vi "Untitled 2.vi"() -> ()   [LabVIEW 2017]
uses:
  JSONtext.lvlib
panel:
  out "Variant out":variant
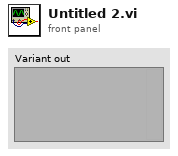
[diagram p1: front panel]
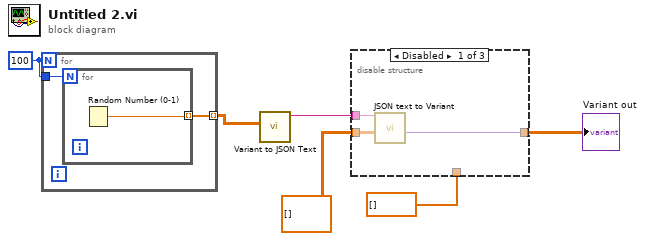
[diagram p0: block diagram]
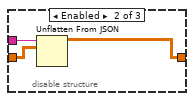
[diagram p2: hidden frame]
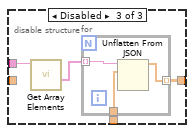
[diagram p3: hidden frame]
diagram:
  w2 = 100
  n1 = for {
    N: w2 -> [_]
    tunnel: [w8] -> w6 mode=indexing
    tunnel: w2 -> [w7]
    n2 = for {
      N: w7 -> [_]
      tunnel: [w9] -> w8 mode=indexing
      n3 = Random Number (0-1)() -> (number: 0 to 1=w9:dbl)
    }
  }
  n4 = call "Variant to JSON Text.vi"("Variant"=w6) -> ("<JSON>"=w5:string)  [unwired: 8 in, 2 out]
  n5 = disable-structure shown="Disabled" {
    disable-tunnel: w5 -> [w12 w15 w19]
    disable-tunnel: dbl[][] [] -> [w11 w14 _]
    disable-tunnel: [w10 w13 w16] -> w3
    disable-tunnel: dbl[] [] -> [_ _ w17]
    frame Disabled {
      n6 = call "JSON text to Variant.vi"("Data Type"=w11, "JSON"=w12) -> ("Variant out"=w10:variant)  [unwired: 8 in, 1 out]
    }
    frame Enabled {
      n7 = Unflatten From JSON(JSON string=w15, type and defaults=w14) -> (value=w13:dbl[][])  [unwired: 5 in, 1 out]
    }
    frame Disabled {
      n8 = call "Get Array Elements.vi"("JSON"=w19) -> ("<JSON>"=w18:string[])  [unwired: 8 in, 2 out]
      n9 = for {
        tunnel: w18 -> [w22] mode=indexing
        tunnel: w17 -> [w21]
        tunnel: [w20] -> w16 mode=indexing
        n10 = Unflatten From JSON(JSON string=w22, type and defaults=w21) -> (value=w20:dbl[])  [unwired: 5 in, 1 out]
      }
    }
  }
  "Variant out" <- w3
